vi "Set Selected Mapping.vi"(8 "error in (no error)":errorcluster, 9 "Index":i32, 10 "Item Names":string[][](array[string]), 11 "Loop Data in":T1) -> (0 "error out":errorcluster, 3 "Loop Data out":T1)   [LabVIEW 2016, in "System Mapping Tool.lvlib"]
uses:
  System Mapping Tool.lvlib
  TypeDefs/Loop Data.ctl
  TypeDefs/UI Refs.ctl
  NationalInstruments.VeriStand.SystemDefinitionAPI
  NationalInstruments.VeriStand.SystemStorageUI
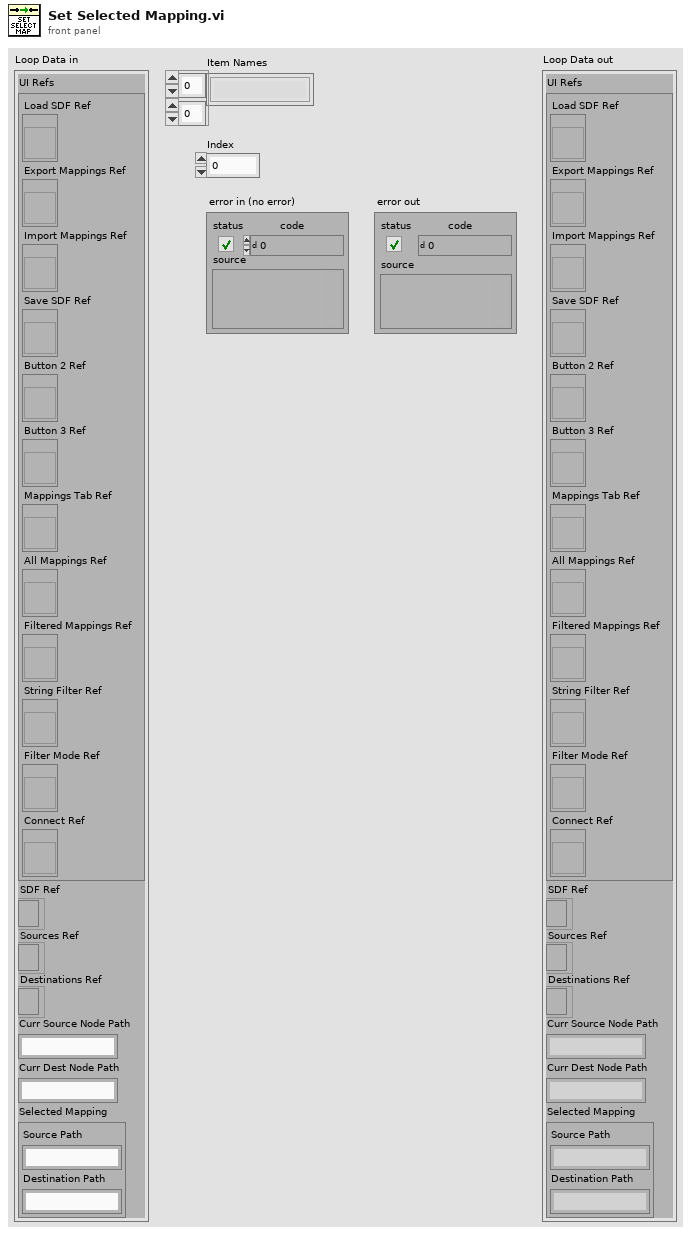
[diagram p1: front panel]
types:
  T1 = typedef "System Mapping Tool.lvlib/Loop Data.ctl" = cluster{"UI Refs":T2, "SDF Ref":refnum<k24>, "Sources Ref":refnum<k24>, "Destinations Ref":refnum<k24>, "Curr Source Node Path":string, "Curr Dest Node Path":string, "Selected Mapping":cluster{"Source Path":string, "Destination Path":string}}
  T2 = typedef "System Mapping Tool.lvlib/UI Refs.ctl" = cluster{"Load SDF Ref":refnum<vi>, "Export Mappings Ref":refnum<vi>, "Import Mappings Ref":refnum<vi>, "Save SDF Ref":refnum<vi>, "Button 2 Ref":refnum<vi>, "Button 3 Ref":refnum<vi>, "Mappings Tab Ref":refnum<vi>, "All Mappings Ref":refnum<vi>, "Filtered Mappings Ref":refnum<vi>, "String Filter Ref":refnum<vi>, "Filter Mode Ref":refnum<vi>, "Connect Ref":refnum<vi>}
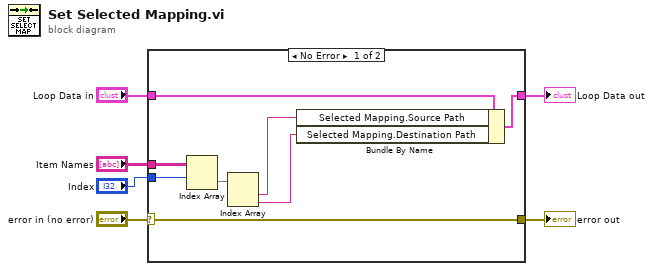
[diagram p0: block diagram]
diagram:
  n1 = case shown="No Error" "error in (no error)" {
    selector: "error in (no error)" -> [w7 w16]
    tunnel: [w7 w16] -> w5
    tunnel: "Loop Data in" -> [w14 w15]
    tunnel: [w13 w15] -> w3
    tunnel: "Item Names" -> [w12 _]
    tunnel: "Index" -> [w11 _]
    frame No Error {
      n2 = Index Array(array=w12, index (row)=w11) -> (element=w10:string[])  [unwired: 1 in]
      n3 = Index Array(array=w10) -> (element #1=w9:string, element #2=w8:string)  [unwired: 2 in]
      n4 = Bundle By Name(cluster=w14, "Selected Mapping.Source Path"=w9, "Selected Mapping.Destination Path"=w8) -> (w13:T1)
    }
    frame Error {
    }
  }
  "Loop Data out" <- w3
  "error out" <- w5
